vi "tele_threashold.vi"() -> ()   [LabVIEW 2012, in "BlockParty4150.lvrbt"]
uses:
  BlockParty4150.lvrbt
  <vilib>/NXT/Hardware/Plugins/Tetrix DC Motor/TetrixDCMotorAddress.ctl
  <vilib>/NXT/LegoClasses/BrickReference/BrickReference.lvclass
  <vilib>/NXT/Subs/LVHSConnector.ctl
  <vilib>/NXT/NXTIO Xnodes/NXTIONodeSubVIs/TETRIX IO Move DC Motors.vi
  <vilib>/NXT/NXTIO Xnodes/NXTIOXNode/NXTIO.xnode
  <vilib>/NXT/NXTIO Xnodes/AddressXNode/NXTIOAddress.xnode
  <vilib>/NXT/NXTIO Xnodes/NXTIONodeSubVIs/TETRIX IO Check Battery.vi
  <vilib>/NXT/NXTIO Xnodes/NXTIONodeSubVIs/TETRIX IO Stop DC Motors.vi
  <vilib>/NXT/Dual Mode Library/Display/drawNumber.vi
  <vilib>/FTC/FTC Calculate Drive Power - Tank.vi
panel:
  out "Enabled?":enum16{"Disabled", "Enabled"}(ring)
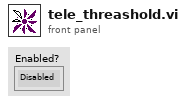
[diagram p1: front panel]
types:
  T1 = typedef "LVHSConnector.ctl" = refnum<class "BrickReference.lvclass">
  T2 = typedef "TetrixDCMotorAddress.ctl" = i16
  T3 = cluster{"TetrixDCMotor":T2, "TetrixDCMotor 2":T2}
  T4 = typedef "FTC ControllerState.ctl" = cluster{"Left X":i8, "Left Y":i8, "Right X":i8, "Right Y":i8, "Button Encoding 9-12":u8, "Button Encoding 1-8":u8, "POV":T5}
  T5 = typedef "FTC POVState.ctl" = i8
  T6 = typedef "FTC ButtonEventType.ctl" = enum16{"Pressed", "Released"}
  T7 = cluster{"Button ID":enum16{"None", "Button 1", "Button 2", "Button 3", "Button 4", "Button 5", "Button 6", "Button 7", "Button 8", "Button 9", "Button 10", "Button 11", "Button 12", "POV Up", "POV Up Right", "POV Right", "POV Down Right", "POV Down", "POV Down Left", "POV Left", "POV Up Left"}, "Event Type":T6}[]
  T8 = enum16{"None", "Button 1", "Button 2", "Button 3", "Button 4", "Button 5", "Button 6", "Button 7", "Button 8", "Button 9", "Button 10", "Button 11", "Button 12", "POV Up", "POV Up Right", "POV Right", "POV Down Right", "POV Down", "POV Down Left", "POV Left", "POV Up Left"}
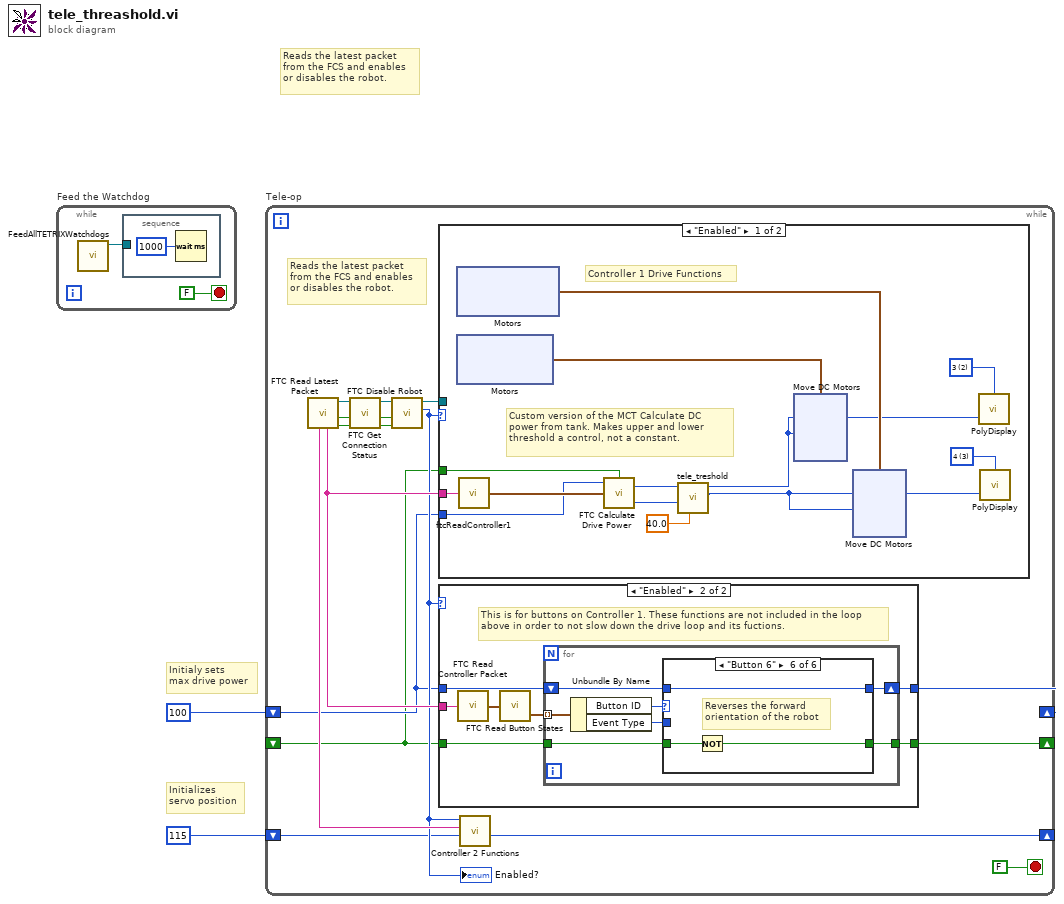
[diagram p0: block diagram]
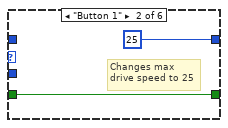
[diagram p4: hidden frame]
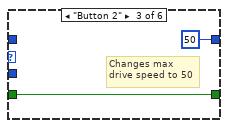
[diagram p5: hidden frame]
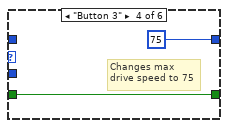
[diagram p6: hidden frame]
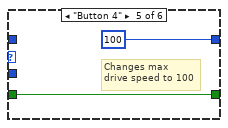
[diagram p7: hidden frame]
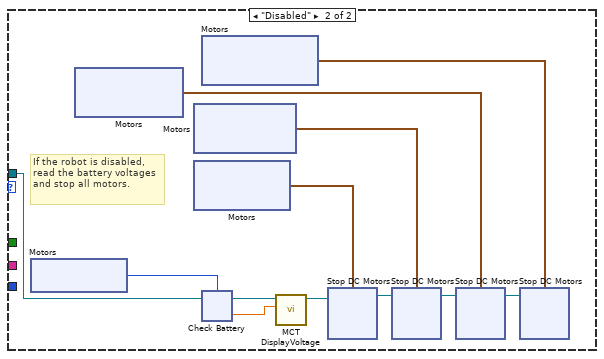
[diagram p8: hidden frame]
diagram:
  # "Initializes \nservo position"
  # "Initialy sets\nmax drive power"
  # "Reads the latest packet\nfrom the FCS and enables\nor disables the robot."
  n1 = while "Feed the Watchdog" {
    stop <- FALSE stop-if-true
    n2 = call <vilib>:"FeedAllTETRIXWatchdogs.vi"() -> ("NXT"=w3:T1)  [unwired: 11 in]
    n3 = stacked-sequence {
      tunnel: w3 -> [_]
      frame #0 {
        n4 = Wait (ms)(milliseconds to wait=u32 1000) -> ()  [unwired: 1 out]
      }
    }
  }
  n5 = while "Tele-op" {
    shift-right: [w14] -> _
    shift-left: i8 100 ("Power Level (50)") -> [w8]
    shift-right: [w13] -> _
    shift-left: _ -> [w6]
    shift-right: [w7] -> _
    shift-left: u8 115 ("f") -> [w9]
    stop <- FALSE stop-if-true
    # "Reads the latest packet\nfrom the FCS and enables\nor disables the robot."
    n6 = call <vilib>:"FTC Read Latest Packet.vi"() -> ("Packet Received?"=w21:bool, "Stopped?"=w19:bool, "NXT"=w20:T1, "Controller 1"=w12:string, "Controller 2"=w11:string)  [unwired: 6 in, 1 out]
    n7 = call <vilib>:"FTC Get Connection Status.vi"("Packet Received?"=w21, "Stopped?"=w19, "NXT"=w20) -> ("Online?"=w16:bool, "Stopped?"=w17:bool, "NXT"=w18:T1)  [unwired: 5 in]
    n8 = call <vilib>:"FTC Disable Robot.vi"("Online?"=w16, "Stopped?"=w17, "NXT"=w18) -> ("Enabled?"=w10:enum16{"Disabled", "Enabled"}, "NXT"=w15:T1)  [unwired: 3 in]
    "Enabled?" <- w10
    n9 = case "disableCase" shown="\"Enabled\"" w10 {
      tunnel: w12 -> [w64 _]
      tunnel: w15 -> [_ w98]
      tunnel: w8 -> [w60 _]
      tunnel: w6 -> [w59 _]
      frame "Enabled" {
        w57 = i16 3 items=["1", "2", "3", "4", "5", "6", "7", "8"] ("Line")
        w58 = i16 2 items=["1", "2", "3", "4", "5", "6", "7", "8"] ("Line")
        # "Controller 1 Drive Functions"
        # "Custom version of the MCT Calculate DC power from tank. Makes upper and lower threshold a control, not a constant."
        n10 = xnode ("Motors")() -> ("Motor"=w63:cluster{"TetrixDCMotor":T2, "TetrixDCMotor":T2})
        n11 = xnode ("Motors")() -> ("Motor"=w62:cluster{"TetrixDCMotor":T2, "TetrixDCMotor":T2})
        n12 = call "ftcReadController1"("Packet"=w64) -> ("Controller State"=w61:T4)  [unwired: 4 in]
        n13 = call-poly <vilib>:"FTC Calculate Drive Power.vi"("Reverse"=w59, "Controller State"=w61, "Power Level (50)"=w60) -> ("Right Motor Power"=w53:i8, "Left Motor Power"=w54:i8)  [unwired: 1 in]
        n14 = call "tele_treshold.vi"("lower limit"=40.0, "Right in"=w53, "Left in"=w54) -> ("Right out"=w56:i8, "Left out"=w55:i8)  [unwired: 7 in]
        n15 = xnode ("Move DC Motors")("Power/Speed 2"=w55, "Power/Speed 1"=w55, "Motors"=w62) -> ()  [unwired: 1 in, 1 out]
        n16 = xnode ("Move DC Motors")("Power/Speed 2"=w56, "Power/Speed 1"=w56, "Motors"=w63) -> ()  [unwired: 1 in, 1 out]
        n17 = call-poly <vilib>:"PolyDisplay.vi"("number"=w55, "Line"=w58) -> ()  [unwired: 2 in, 1 out]
        n18 = call-poly <vilib>:"PolyDisplay.vi"("number"=w56, "Line"=w57) -> ()  [unwired: 2 in, 1 out]
      }
      frame "Disabled" {
        # "If the robot is disabled, read the battery voltages and stop all motors."
        n19 = xnode ("Motors")() -> ("Motor"=w97:T2)
        n20 = xnode "Motors"() -> ("Motor"=w90:cluster{"TetrixDCMotor":T2, "TetrixDCMotor":T2})
        n21 = xnode "Motors"() -> ("Motor"=w92:cluster{"TetrixDCMotor":T2, "TetrixDCMotor":T2})
        n22 = xnode "Motors"() -> ("Motor"=w94:cluster{"TetrixDCMotor":T2, "TetrixDCMotor":T2})
        n23 = xnode "Motors"() -> ("Motor"=w88:cluster{"TetrixDCMotor":T2, "TetrixDCMotor":T2})
        n24 = xnode ("Check Battery")("Motors"=w97, "NXT"=w98) -> ("Voltage 1"=w96:sgl, "NXT"=w95:T1)
        n25 = call <vilib>:"MCT DisplayVoltage.vi"("Motor Voltage"=w96, "NXT"=w95) -> ("NXT"=w93:T1)  [unwired: 9 in]
        n26 = xnode "Stop DC Motors"("Motors"=w94, "NXT"=w93) -> ("NXT"=w91:T1)
        n27 = xnode "Stop DC Motors"("Motors"=w92, "NXT"=w91) -> ("NXT"=w89:T1)
        n28 = xnode "Stop DC Motors"("Motors"=w90, "NXT"=w89) -> ("NXT"=w87:T1)
        n29 = xnode "Stop DC Motors"("Motors"=w88, "NXT"=w87) -> ()  [unwired: 1 out]
      }
    }
    n30 = case shown="\"Enabled\"" w10 {
      tunnel: w12 -> [_ w31]
      tunnel: [w24 w28] -> w14
      tunnel: w8 -> [w24 w27]
      tunnel: [w23 w26] -> w13
      tunnel: w6 -> [w23 w25]
      frame "Disabled", Default {
      }
      frame "Enabled" {
        # "This is for buttons on Controller 1. These functions are not included in the loop above in order to not slow down the drive loop and its fuctions."
        n31 = call <vilib>:"FTC Read Controller Packet.vi"("Packet"=w31) -> ("Controller State"=w30:T4)  [unwired: 4 in]
        n32 = call <vilib>:"FTC Read Button States.vi"("Controller State"=w30) -> ("Button Events"=w29:T7)  [unwired: 2 in, 1 out]
        n33 = for {
          tunnel: w29 -> [w38] mode=indexing
          tunnel: [w33] -> w26
          tunnel: w25 -> [w32]
          shift-right: [w35] -> w28
          shift-left: w27 -> [w34]
          n34 = Unbundle By Name(w38) -> ("Button ID"=w37:T8, "Event Type"=w36:T6)
          n35 = case shown="\"Button 6\"" w37 {
            tunnel: w36 -> [_ _ _ _ _ _]
            tunnel: [w40 i8 25 ("Power Level (50)") i8 50 ("Power Level (50)") i8 75 ("Power Level (50)") i8 100 ("Power Level (50)") w51] -> w35
            tunnel: w34 -> [w40 _ _ _ _ w51]
            tunnel: [w39 w41 w43 w45 w47 w50] -> w33
            tunnel: w32 -> [w39 w41 w43 w45 w47 w49]
            frame "None", Default {
            }
            frame "Button 1" {
              # "Changes max\ndrive speed to 25"
            }
            frame "Button 2" {
              # "Changes max\ndrive speed to 50"
            }
            frame "Button 3" {
              # "Changes max\ndrive speed to 75"
            }
            frame "Button 4" {
              # "Changes max\ndrive speed to 100"
            }
            frame "Button 6" {
              # "Reverses the forward\norientation of the robot"
              n36 = Not(x=w49) -> (.not. x?=w50:bool)
            }
          }
        }
      }
    }
    n37 = call "Controller 2 Functions.vi"("Servo In"=w9, "Controller in"=w11, "Enabled?"=w10) -> ("Servo Out"=w7:u8)  [unwired: 8 in]
  }
